vi "SSL_CTX_set_options.vi"(8 "error in (no error)":errorcluster, 10 "Options":T1=50462720 items=["None"=0, "NO_SSLv2|v3|COMPRESSION"=50462720, "SSL_OP_NO_COMPRESSION"=131072, "SSL_OP_NO_SSLv2"=16777216, "SSL_OP_NO_SSLv3"=33554432, "SSL_OP_NO_TLSv1"=67108864, "SSL_OP_NO_TLSv1_2"=134217728, "SSL_OP_NO_TLSv1_1"=268435456], 11 "SSL-Context in":refnum<class "SSL-Context.lvclass">) -> (0 "error out":errorcluster, 3 "SSL-Context out":refnum<class "SSL-Context.lvclass">)   [LabVIEW 2013, in "OpenSSL Socket.lvlib" / "SSL-Context.lvclass"]
uses:
  SSL-Context.lvclass
  SSL Options.ctl
  SSL-Lib/SSL-Lib.lvclass/SSL-Lib.ctl
  SSL-Context.lvclass/SSL-Context.ctl
  SSL-Lib/Read SSL Library Path.vi
  Read Handle.vi
  SSL-Lib/SSL-Lib.lvclass
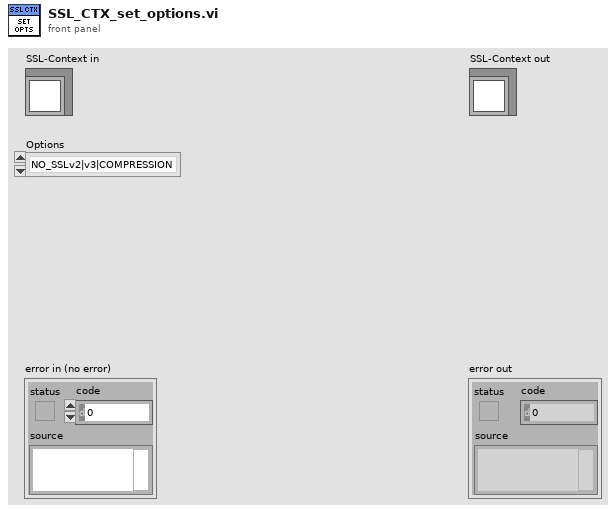
[diagram p1: front panel]
types:
  T1 = typedef "OpenSSL Socket.lvlib/SSL-Context.lvclass/SSL Options.ctl" = i32
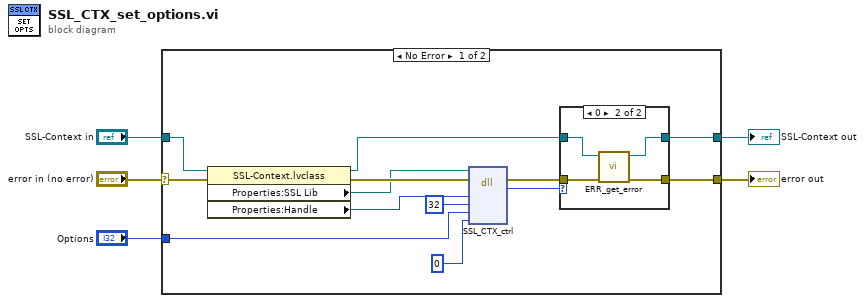
[diagram p0: block diagram]
diagram:
  n1 = case shown="No Error" "error in (no error)" {
    selector: "error in (no error)" -> [w18 w26]
    tunnel: [w6 w26] -> w4
    tunnel: [w10 w25] -> w2
    tunnel: "SSL-Context in" -> [w16 w25]
    tunnel: "Options" -> [w7 _]
    frame No Error {
      n2 = property class="SSL-Context.lvclass"(reference=w16, error in=w18) -> (reference out=w12:refnum<class "SSL-Context.lvclass">, error out=w17:errorcluster, "Properties:SSL Lib"=w15:path, "Properties:Handle"=w14:u64)
      n3 = dll-call lib="C:/Program Files (x86)/National Instruments/Shared/nissl/NIssleay32.dll" fn="SSL_CTX_ctrl"(path in=w15, error in=w17, "SSL_CTX"=w14, "cmd"=32 ("arg2"), "larg"=w7, "parg"=0 ("arg2")) -> (error out=w13:errorcluster, "return type"=w11:i32)  [unwired: 5 in, 1 out]
      n4 = case shown="0" w11 {
        tunnel: w13 -> [w20 w24]
        tunnel: w12 -> [w19 w23]
        tunnel: [w19 w22] -> w10
        tunnel: [w20 w21] -> w6
        frame Default {
        }
        frame 0 {
          n5 = call "ERR_get_error.vi"("error in (no error)"=w24, "SSL-Lib in"=w23) -> ("error out"=w21:errorcluster, "SSL-Lib out"=w22:refnum<class "SSL-Context.lvclass">)  [unwired: 8 in]
        }
      }
    }
    frame Error {
    }
  }
  "error out" <- w4
  "SSL-Context out" <- w2
